vi "Configure Trigger (Glitch).vi"(0 "VISA resource name":refnum<visa-resource-name>, 1 "Trigger Width (500E-12s)":dbl=5e-10, 2 "Polarity (0:Positive)":u16(ring) items=["Positive", "Negative", "Either"], 3 "Trigger Event (0:A Event)":u16(ring) items=["A Event", "B Event"], 5 "Source (0:Channel1)":u16(ring) items=["Channel1", "Channel2", "Channel3", "Channel4", "Digital Channel0", "Digital Channel1", "Digital Channel2", "Digital Channel3", "Digital Channel4", "Digital Channel5", "Digital Channel6", "Digital Channel7", "Digital Channel8", "Digital Channel9", "Digital Channel10", "Digital Channel11", "Digital Channel12", "Digital Channel13", "Digital Channel 14", "Digital Channel 15"], 7 "Trigger Level (0)":dbl, 9 "Trigger Condition (0:Less Than)":u16(ring) items=["Less Than", "Greater Than"], 11 "error in (no error)":errorcluster, 12 "Trigger If Glitch (0:Occurs)":u16(ring) items=["Occurs", "Logic", "Bus"]) -> (4 "VISA resource name out":refnum<visa-resource-name>, 6 "Trigger Event Out":u16(ring) items=["A Event", "B Event"], 15 "error out":errorcluster)   [LabVIEW 2011, in "Tektronix 7000 Series.lvlib"]
doc: "Configures Glitch trigger settings for an oscilloscope.A glitch occurs when the oscilloscope detects a pulse width that is less than or a greater than a specified glitch duration.\n\nTDS5000 ,TDS5000B,TDS6000 ,CSA7000 and TDS7000 series oscilloscopes don't support B Glitch Trigger."
uses:
  Tektronix 7000 Series.lvlib
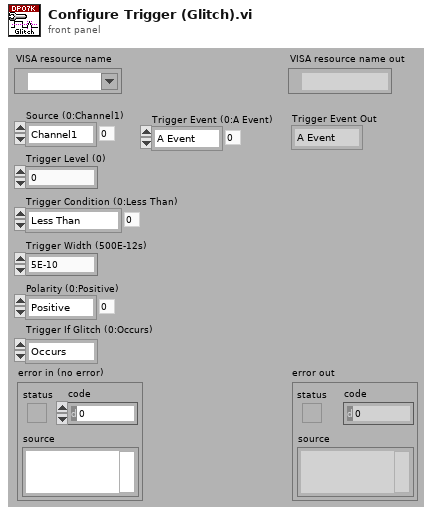
[diagram p1: front panel]
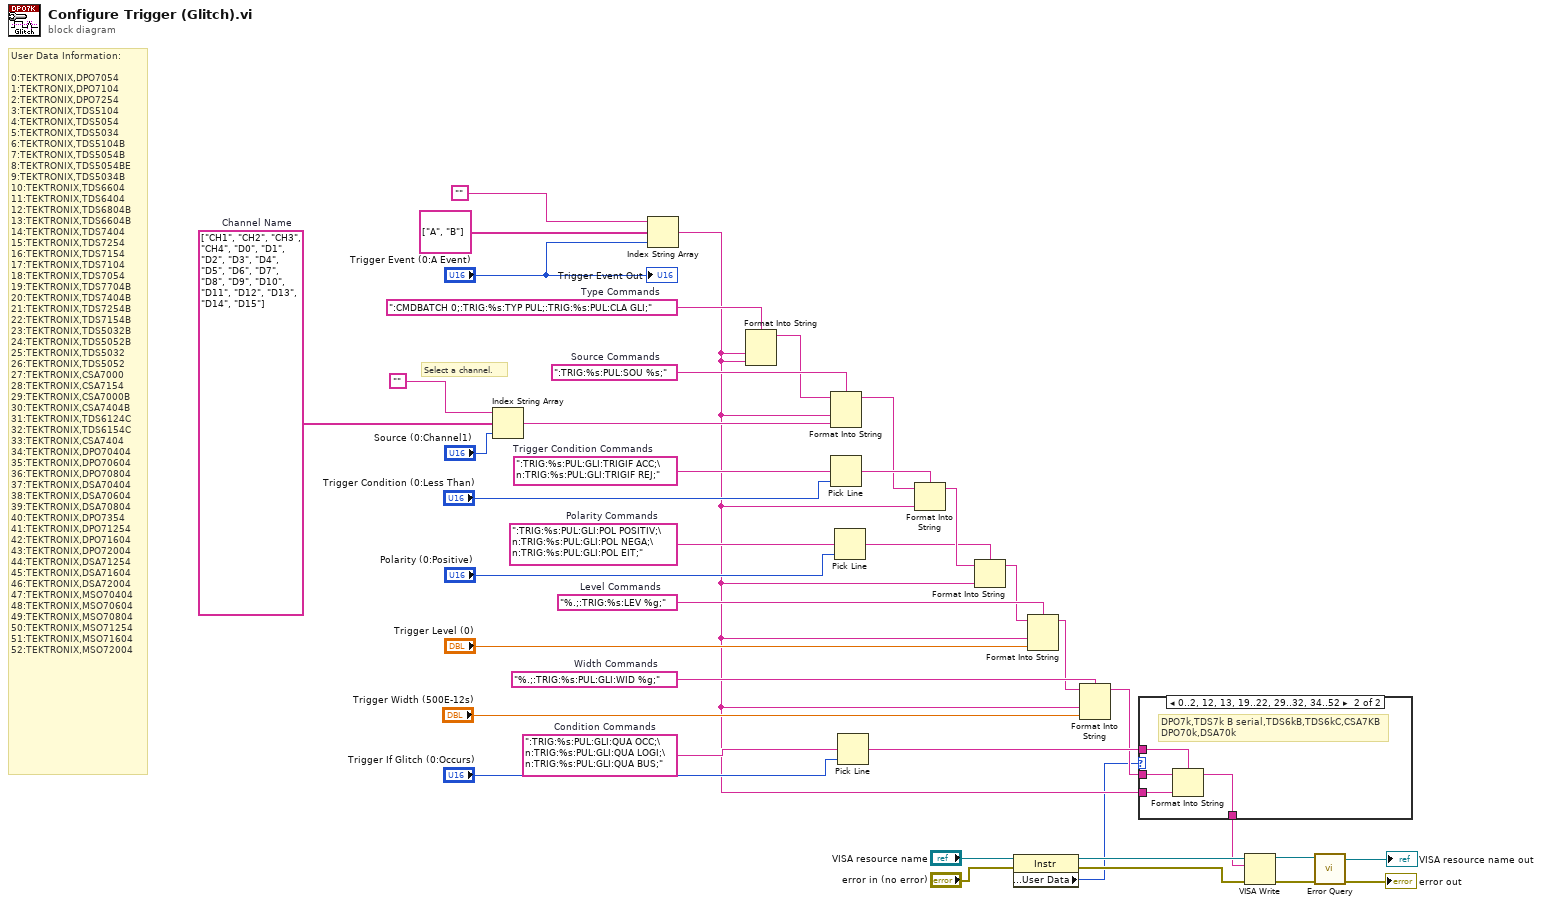
[diagram p0: block diagram]
diagram:
  w21 = ":TRIG:%s:PUL:GLI:QUA OCC;\n:TRIG:%s:PUL:GLI:QUA LOGI;\n:TRIG:%s:PUL:GLI:QUA BUS;"  # Condition Commands
  w22 = ":TRIG:%s:PUL:GLI:POL POSITIV;\n:TRIG:%s:PUL:GLI:POL NEGA;\n:TRIG:%s:PUL:GLI:POL EIT;"  # Polarity Commands
  w24 = ":TRIG:%s:PUL:GLI:TRIGIF ACC;\n:TRIG:%s:PUL:GLI:TRIGIF REJ;"  # Trigger Condition Commands
  w23 = "%.;:TRIG:%s:PUL:GLI:WID %g;"  # Width Commands
  w25 = "%.;:TRIG:%s:LEV %g;"  # Level Commands
  w26 = ":TRIG:%s:PUL:SOU %s;"  # Source Commands
  w19 = ":CMDBATCH 0;:TRIG:%s:TYP PUL;:TRIG:%s:PUL:CLA GLI;"  # Type Commands
  w39 = string[] ["CH1", "CH2", "CH3", "CH4", "D0", "D1", "D2", "D3", "D4", "D5", "D6", "D7", "D8", "D9", "D10", "D11", "D12", "D13", "D14", "D15"]  # Channel Name
  # "User Data Information:\n\n0:TEKTRONIX,DPO7054\n1:TEKTRONIX,DPO7104\n2:TEKTRONIX,DPO7254\n3:TEKTRONIX,TDS5104\n4:TEKTRONIX,TDS5054\n5:TEKTRONIX,TDS5034\n6:TEKTRONIX,TDS5104B\n7:TEKTRONIX,TDS5054B\n8:TEKTRONIX,TDS5054BE\n9:TEKTRONIX,TDS5034B\n10:TEKTRONIX,TDS6604\n11:TEKTRONIX,TDS6404\n12:TEKTRONIX,TDS6804B\n13:TEKTRONIX,TDS6604B\n14:TEKTRONIX,TDS7404\n15:TEKTRONIX,TDS7254\n16:TEKTRONIX,TDS7154\n17:TEKTRONIX,TDS7104\n18:TEKTRONIX,TDS7054\n19:TEKTRONIX,TDS7704B\n20:TEKTRONIX,TDS7404B\n21:TEKTRONIX,TDS7254B\n22:TEKTRONIX,TDS7154B\n23:TEKTRONIX,TDS5032B\n24:TEKTRONIX,TDS5052B\n25:TEKTRONIX,TDS5032\n26:TEKTRONIX,TDS5052\n27:TEKTRONIX,CSA7000\n28:TEKTRONIX,CSA7154\n29:TEKTRONIX,CSA7000B\n30:TEKTRONIX,CSA7404B\n31:TEKTRONIX,TDS6124C\n32:TEKTRONIX,TDS6154C\n33:TEKTRONIX,CSA7404\n34:TEKTRONIX,DPO70404\n35:TEKTRONIX,DPO70604\n36:TEKTRONIX,DPO70804\n37:TEKTRONIX,DSA70404\n38:TEKTRONIX,DSA70604\n39:TEKTRONIX,DSA70804\n40:TEKTRONIX,DPO7354\n41:TEKTRONIX,DPO71254\n42:TEKTRONIX,DPO71604\n43:TEKTRONIX,DPO72004\n44:TEKTRONIX,DSA71254\n45:TEKTRONIX,DSA71604\n46:TEKTRONIX,DSA72004\n47:TEKTRONIX,MSO70404\n48:TEKTRONIX,MSO70604\n49:TEKTRONIX,MSO70804\n50:TEKTRONIX,MSO71254\n51:TEKTRONIX,MSO71604\n52:TEKTRONIX,MSO72004"
  # "Select a channel."
  n1 = Index String Array(1:"Source (0:Channel1)", 2:w39, 3:"" ("Empty String Constant")) -> (0:w18:string)
  n2 = Index String Array(1:"Trigger Event (0:A Event)", 2:string[] ["A", "B"], 3:"" ("Empty String Constant")) -> (0:w9:string)
  n3 = Format Into String(format string=w19, w9, w9) -> (resulting string=w17:string)  [unwired: 2 in, 1 out]
  n4 = Format Into String(format string=w26, initial string=w17, w9, w18) -> (resulting string=w15:string)  [unwired: 1 in, 1 out]
  n5 = Pick Line(multi-line string=w24, line index="Trigger Condition (0:Less Than)") -> (output string=w16:string)  [unwired: 1 in]
  n6 = Pick Line(multi-line string=w22, line index="Polarity (0:Positive)") -> (output string=w13:string)  [unwired: 1 in]
  n7 = Pick Line(multi-line string=w21, line index="Trigger If Glitch (0:Occurs)") -> (output string=w12:string)  [unwired: 1 in]
  n8 = Format Into String(format string=w16, initial string=w15, w9) -> (resulting string=w14:string)  [unwired: 1 in, 1 out]
  n9 = Format Into String(format string=w13, initial string=w14, w9) -> (resulting string=w8:string)  [unwired: 1 in, 1 out]
  n10 = property class="Instr"(reference="VISA resource name", error in="error in (no error)") -> (reference out=w4:refnum<visa-resource-name>, error out=w3:errorcluster, "General Settings:User Data"=w2:u32)
  n11 = Format Into String(format string=w25, initial string=w8, w9, "Trigger Level (0)") -> (resulting string=w20:string)  [unwired: 1 in, 1 out]
  n12 = Format Into String(format string=w23, initial string=w20, w9, "Trigger Width (500E-12s)") -> (resulting string=w7:string)  [unwired: 1 in, 1 out]
  n13 = case shown="0..2, 12, 13, 19..22, 29..32, 34..52" w2 {
    tunnel: w12 -> [_ w44]
    tunnel: w9 -> [_ w43]
    tunnel: w7 -> [w40 w42]
    tunnel: [w40 w41] -> w1
    frame Default {
    }
    frame 0..2, 12, 13, 19..22, 29..32, 34..52 {
      # "DPO7k,TDS7k B serial,TDS6kB,TDS6kC,CSA7KB\nDPO70k,DSA70k"
      n14 = Format Into String(format string=w44, initial string=w42, w43) -> (resulting string=w41:string)  [unwired: 1 in, 1 out]
    }
  }
  n15 = VISA Write(VISA resource name=w4, write buffer=w1, error in (no error)=w3) -> (VISA resource name out=w33:refnum<visa-resource-name>, error out=w32:errorcluster)  [unwired: 1 out]
  n16 = call "Error Query.vi"("error in (no error)"=w32, "VISA resource name"=w33) -> ("error out"=→"error out":errorcluster, "VISA resource name out"=→"VISA resource name out":refnum<visa-resource-name>)  [unwired: 6 in, 2 out]
  "Trigger Event Out" <- "Trigger Event (0:A Event)"
